vi "Robot Global Data.vi"() -> ()   [LabVIEW 2013]
doc: "This global VI can contain as many global variables as you need. Place a control on the panel, give it a good name. To read or write to it from a VI, drag the icon to the diagram of that VI. You can also drag from the project. Click on the node to change which global you access. You shouldn't have multiple locations writing to a global or it will cause a race-condition."
uses:
  <vilib>/Rock Robotics/WPI/Camera/WPI_CameraImageSize.ctl
  <vilib>/Rock Robotics/WPI/DriverStation/WPI_DriverStationRobotMode2.ctl
panel:
  in  "AutonomousLoop":bool
  in  "No Kicker":bool
  in  "EndItEndItAll":bool
  in  "Intake":T1(ring)
  out "LeftLock":dbl
  out "RightLock":dbl
  out "ZTrim":dbl
  in  "Driver8":bool
  in  "EncoderLock":bool
  in  "GyroLock":bool
  in  "DoNotDisturb":bool
  in  "PickupOnly":bool
  out "IntakePot":dbl
  out "KickerPot":dbl
  in  "IntakeUp":dbl=0.284502694
  in  "Operator10":bool
  in  "ResetEncoders":bool
  in  "Autonomous":bool
  out "OperatorY":dbl
  in  "Operator9":bool
  in  "Operator6":bool
  in  "Operator3":bool
  in  "Operator2":bool
  in  "Operator1":bool
  in  "Operator7":bool
  in  "DesiredDriveDistance":dbl=62.0
  in  "DrivingPID":bool
  in  "KickerPID":bool
  in  "KickerSetpoint":dbl=4.0
  in  "KickerP":dbl=0.45
  out "InchesRight":dbl=-0.0
  out "InchesLeft":dbl
  in  "Iterator":dbl
  in  "Intake Setpoint":dbl
  in  "IntakePID":bool
  in  "Intake State":T2(ring)
  in  "SpinShaft":bool
  out "DriveY":dbl
  out "DriveX":dbl
  in  "Robot Mode":T3
  in  "LED toggle rate (ms)":u32=20
  in  "image size":T4=enum."320x240"
  in  "Enable Vision":bool
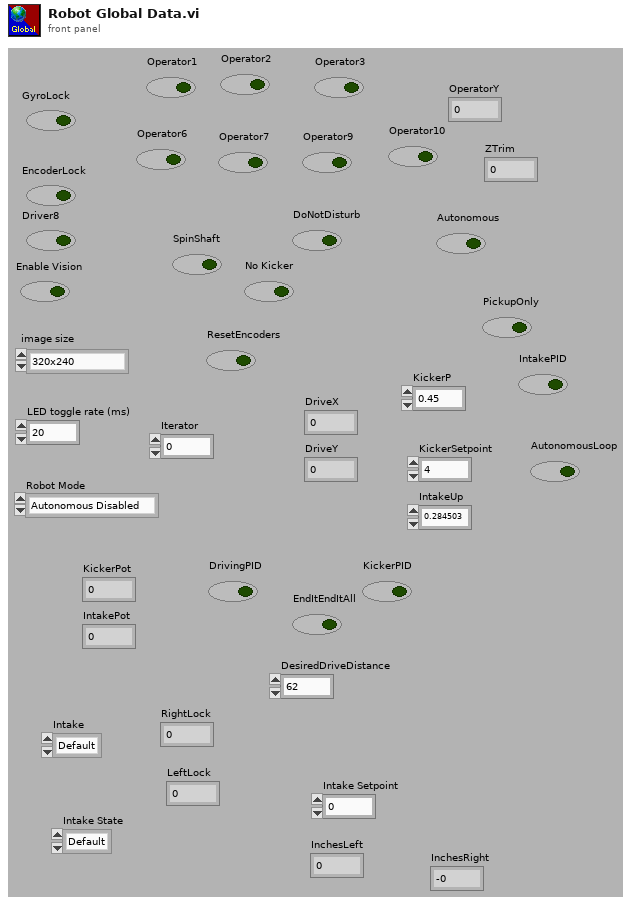
[diagram p1: front panel]
types:
  T1 = enum16{"Default", "Set", "Pickup", "Place", "KickerUp", "Rest", "Kick", "End"}
  T2 = enum16{"Default", "Set", "Pickup", "Place", "KickerUp", "Rest", "Kick", "Rest2", "Up", "End"}
  T3 = typedef "WPI_DriverStationRobotMode2.ctl" = enum16{"Autonomous Disabled", "Autonomous Enabled", "Teleop Disabled", "Teleop Enabled", "Timeout", "Finish", "Test Disabled", "Test Enabled"}
  T4 = typedef "WPI_CameraImageSize.ctl" = enum16{"640x480", "320x240", "160x120"}
diagram:
